vi "View.vi"() -> (0 "Boolean 2":bool)   [LabVIEW 2009]
panel:
  in  "OK":bool
  in  "Boolean":bool
  # "Click OK after making selection"
  # "Measure"
  # "Preview"
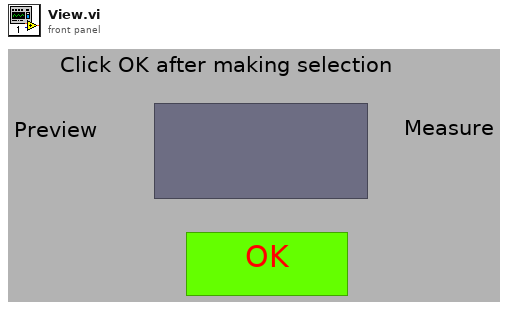
[diagram p1: front panel]
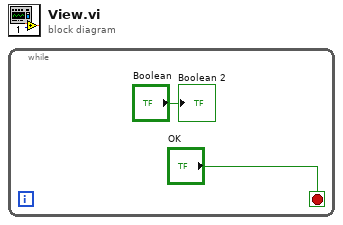
[diagram p0: block diagram]
diagram:
  n1 = while {
    stop <- "OK" stop-if-true
    "Boolean 2" <- "Boolean"
  }
